vi "Set Port Number.vi"(8 "error in":errorcluster, 10 "port number":u16, 11 "port":T1 format="%.0x") -> (0 "error out":errorcluster, 3 "port out":T1 format="%.0x")   [LabVIEW 2020, in "AIM MIL-STD-1553 Scripting.lvlib"]
doc: "Sets the <b>port number</b> for the specified <b>port</b>."
uses:
  AIM MIL-STD-1553 Scripting.lvlib
  <vilib>/NI VeriStand/Custom Device API/Custom Device Item Ref.ctl
  Constants.vi
  <vilib>/NI VeriStand/Custom Device API/Set Item Property (U16).vi
  <vilib>/NI VeriStand/Custom Device API/Custom Device API.lvlib
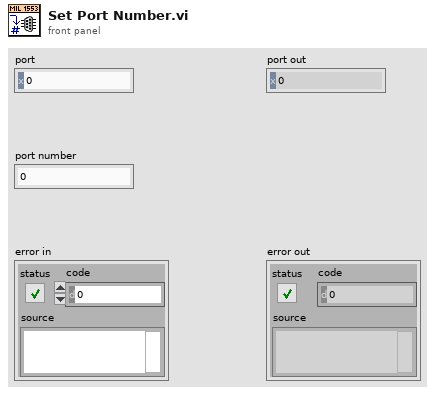
[diagram p1: front panel]
types:
  T1 = typedef "Custom Device API.lvlib/Custom Device Item Ref.ctl" = u64
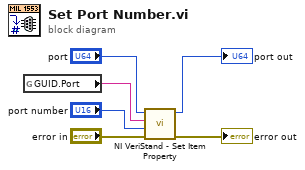
[diagram p0: block diagram]
diagram:
  n1 = global read "Constants.vi" "GUID.Port"() -> (w1:string)
  n2 = call-poly <vilib>:"NI VeriStand - Set Item Property.vi"("error in (no error)"="error in", "Value"="port number", "Property Name"=w1, "Item Ref in"="port") -> ("error out"=→"error out":errorcluster, "Item Ref out"=→"port out":T1)  [unwired: 5 in, 1 out]
